vi "TestSubject.vi"(1 "Text Ring":u16(ring), 9 "Listbox":i32(listbox) caption="ddd", 11 "Boolean IN":bool) -> (3 "Boolean OUT":bool)   [LabVIEW 2025]
uses:
  System.Windows.Forms
  <vilib>/addons/_XControls/Waveforms with Cursors/Waveforms with Cursors.xctl
panel:
  out "Waveforms with Cursors":waveform(dbl)[](xcontrol)
  in  "PictureBox":refnum<k24>(container)
  in  "TCP Network Connection Refnum":refnum<k5>
  in  "stop":bool
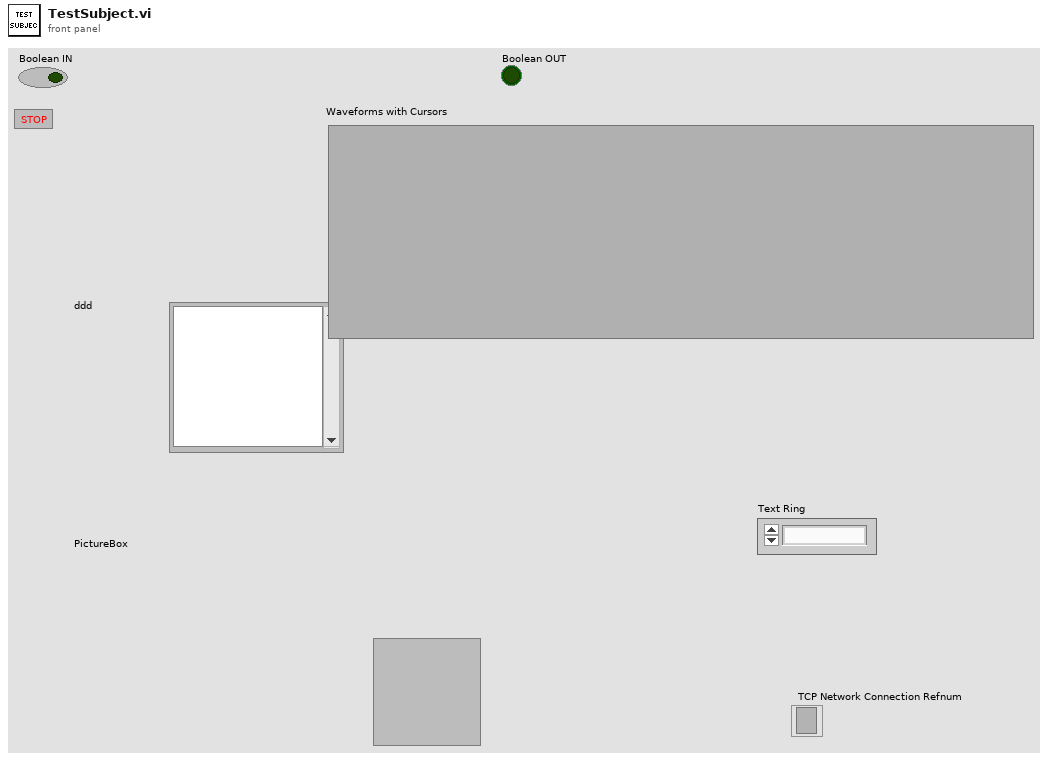
[diagram p1: front panel]
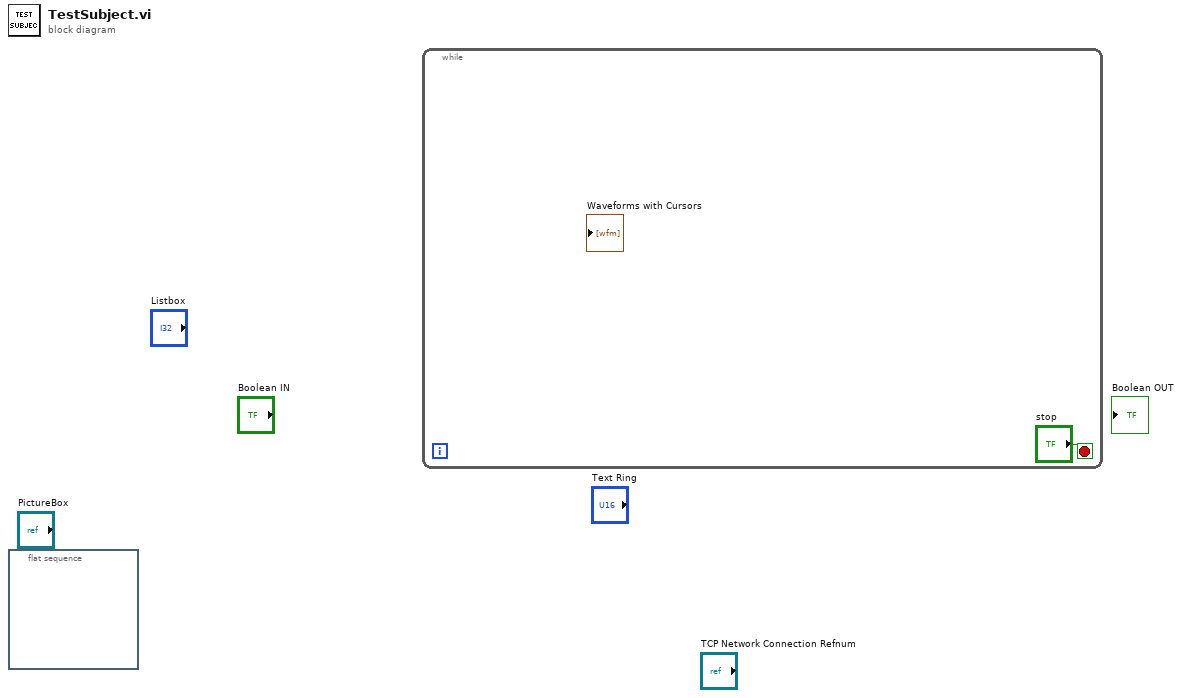
[diagram p0: block diagram]
diagram:
  n1 = flat-sequence {
    frame #0 {
    }
  }
  n2 = while {
    stop <- "stop" stop-if-true
  }
